vi "fgv_stop-point_config.vi"(7 "cmd":enum16{"read", "write"}(ring), 11 "config value":cluster{"stop distance":dbl, "Stop delay":dbl}={"stop distance"=1.0, "Stop delay"=5.0}) -> (3 "config value out":cluster{"stop distance":dbl, "Stop delay":dbl})   [LabVIEW 2019]
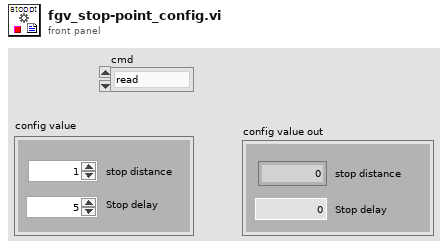
[diagram p1: front panel]
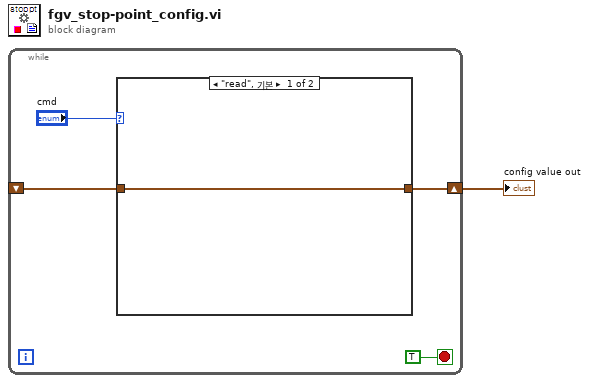
[diagram p0: block diagram]
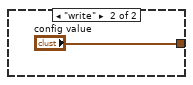
[diagram p2: hidden frame]
diagram:
  n1 = while {
    shift-right: [w3] -> w1
    shift-left: _ -> [w2]
    stop <- TRUE stop-if-true
    n2 = case shown="\"read\", 기본" "cmd" {
      tunnel: [w6 "config value"] -> w3
      tunnel: w2 -> [w6 _]
      frame "read", Default {
      }
      frame "write" {
      }
    }
  }
  "config value out" <- w1
